vi "nPoints Concept - 7 Segment LED.vi"() -> ()   [LabVIEW 2013]
uses:
  <vilib>/DAQmx/write.llb/DAQmx Write (Digital 1D Bool 1Chan 1Samp).vi
  <vilib>/DAQmx/create/channels.llb/DAQmx Create Channel (DO-Digital Output).vi
  <vilib>/DAQmx/miscellaneous.llb/DAQmx Fill In Error Info.vi
panel:
  in  "7 Segment LED":T1
  in  "Count Time (ms)":u32=500
  in  "Count":bool caption="Blink"
  in  "Stop":bool
  # "7 Segment LED"
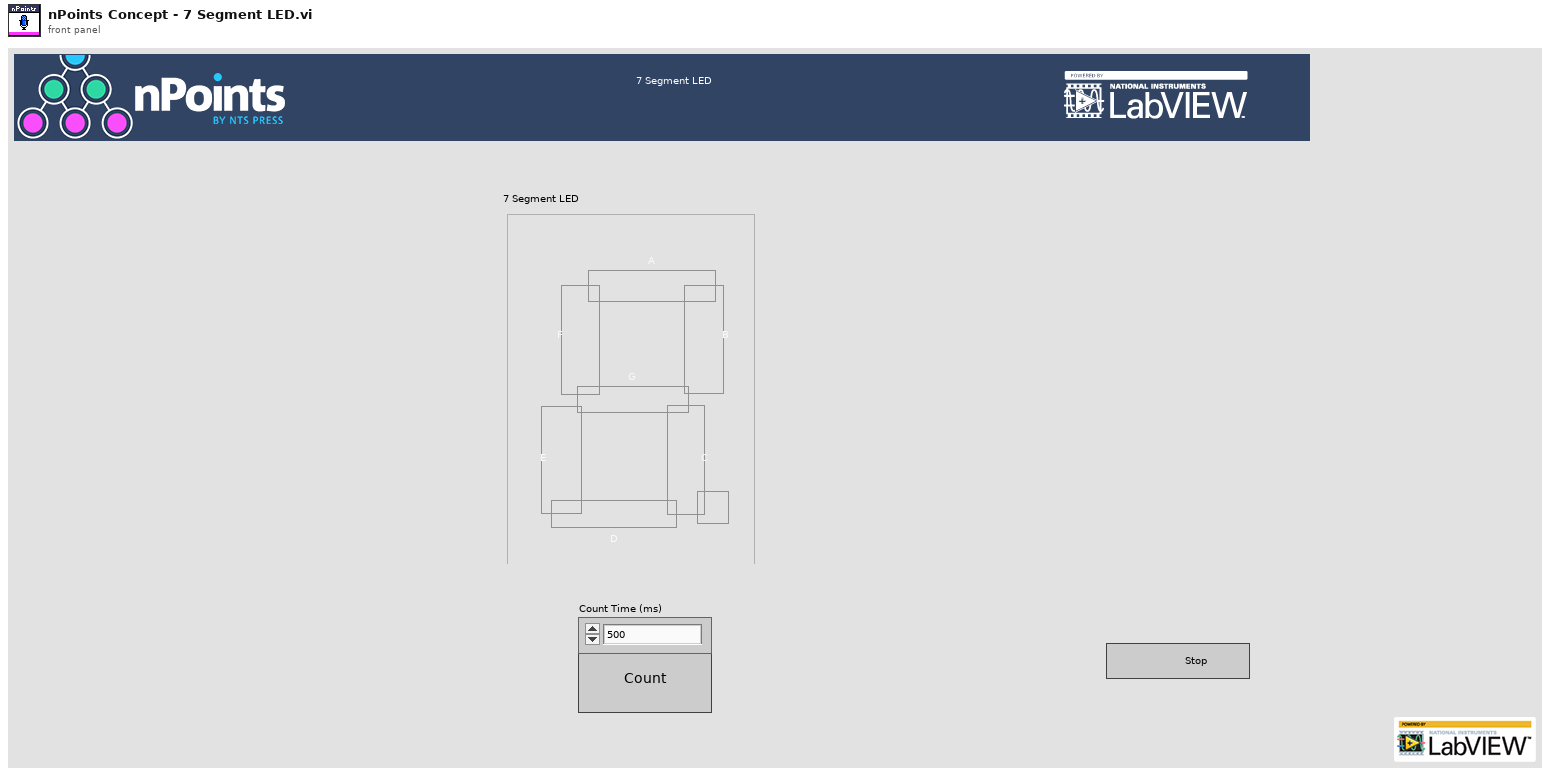
[diagram p1: front panel]
types:
  T1 = cluster{"A":bool, "B":bool, "C":bool, "D":bool, "E":bool, "F":bool, "G":bool, "Dot":bool}
  T2 = cluster{"A":bool, "B":bool, "C":bool, "D":bool, "E":bool, "F":bool, "G":bool, "Dot":bool}[]
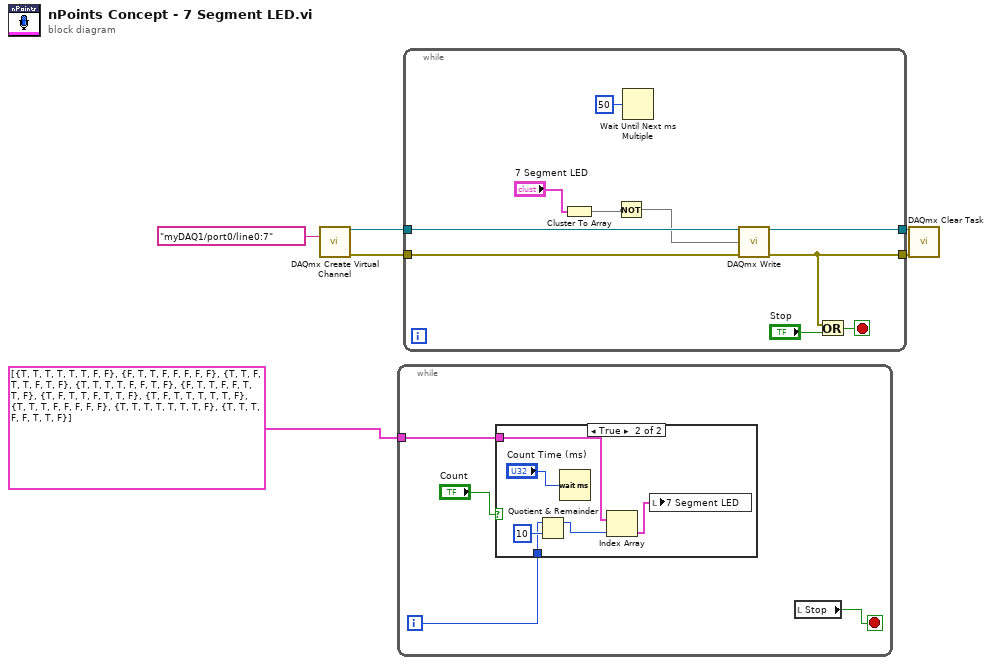
[diagram p0: block diagram]
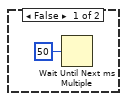
[diagram p2: hidden frame]
diagram:
  n1 = call-poly <vilib>:"DAQmx Create Virtual Channel.vi"("lines"=tag "myDAQ1/port0/line0:7") -> ("task out"=w3:refnum<k21>, "error out"=w4:errorcluster)  [unwired: 13 in]
  n2 = while {
    tunnel: T2 [{"A"=TRUE, "B"=TRUE, "C"=TRUE, "D"=TRUE, "E"=TRUE, "F"=TRUE, "G"=FALSE, "Dot"=FALSE}, {"A"=FALSE, "B"=TRUE, "C"=TRUE, "D"=FALSE, "E"=FALSE, "F"=FALSE, "G"=FALSE, "Dot"=FALSE}, {"A"=TRUE, "B"=TRUE, "C"=FALSE, "D"=TRUE, "E"=TRUE, "F"=FALSE, "G"=TRUE, "Dot"=FALSE}, {"A"=TRUE, "B"=TRUE, "C"=TRUE, "D"=TRUE, "E"=FALSE, "F"=FALSE, "G"=TRUE, "Dot"=FALSE}, {"A"=FALSE, "B"=TRUE, "C"=TRUE, "D"=FALSE, "E"=FALSE, "F"=TRUE, "G"=TRUE, "Dot"=FALSE}, {"A"=TRUE, "B"=FALSE, "C"=TRUE, "D"=TRUE, "E"=FALSE, "F"=TRUE, "G"=TRUE, "Dot"=FALSE}, {"A"=TRUE, "B"=FALSE, "C"=TRUE, "D"=TRUE, "E"=TRUE, "F"=TRUE, "G"=TRUE, "Dot"=FALSE}, {"A"=TRUE, "B"=TRUE, "C"=TRUE, "D"=FALSE, "E"=FALSE, "F"=FALSE, "G"=FALSE, "Dot"=FALSE}, {"A"=TRUE, "B"=TRUE, "C"=TRUE, "D"=TRUE, "E"=TRUE, "F"=TRUE, "G"=TRUE, "Dot"=FALSE}, {"A"=TRUE, "B"=TRUE, "C"=TRUE, "D"=FALSE, "E"=FALSE, "F"=TRUE, "G"=TRUE, "Dot"=FALSE}] ("Array") -> [w7]
    i -> [w10]
    stop <- w9 stop-if-true
    n3 = case shown="True" "Count" {
      tunnel: w10 -> [_ w15]
      tunnel: w7 -> [_ w14]
      frame False {
        n4 = Wait Until Next ms Multiple(millisecond multiple=u32 50) -> ()  [unwired: 1 out]
      }
      frame True {
        n5 = Quotient & Remainder(x=w15, y=10) -> (x-y*floor(x/y)=w12:i32)  [unwired: 1 out]
        n6 = Wait (ms)(milliseconds to wait="Count Time (ms)") -> ()  [unwired: 1 out]
        n7 = Index Array(array=w14, index=w12) -> (element=w13:T1)
        n8 = local write "7 Segment LED"(w13) -> ()
      }
    }
    n9 = local read "Stop"() -> (w9:bool)
  }
  n10 = while {
    tunnel: w4 -> [w24]
    tunnel: w3 -> [w25]
    tunnel: [w23] -> w6
    tunnel: [w22] -> w5
    stop <- w26 stop-if-true
    n11 = Cluster To Array(cluster="7 Segment LED") -> (array=w19:bool[])
    n12 = Not(x=w19) -> (.not. x?=w18:bool[])
    n13 = Wait Until Next ms Multiple(millisecond multiple=u32 50) -> ()  [unwired: 1 out]
    n14 = call-poly <vilib>:"DAQmx Write.vi"("task/channels in"=w25, "data"=w18, "error in"=w24) -> ("task out"=w23:refnum<k21>, "error out"=w22:errorcluster)  [unwired: 10 in, 1 out]
    n15 = Or(x=w22, y="Stop") -> (x .or. y?=w26:bool)
  }
  n16 = call <vilib>:"DAQmx Clear Task.vi"("task in"=w6, "error in"=w5) -> ()  [unwired: 13 in, 1 out]
